vi "TC1001.vi"() -> ()   [LabVIEW 2019]
panel:
  out "ACANMsgBuffer":T1(array[cluster])
  out "初始化的数组 2":T1(array[cluster])
  out "Message&ID":string[](array[string])
  in  "发送":bool
  out "初始化的数组":string[](array[string])
  out "ALLName":string[](array[string])
  out "SignalName":string[][](array[string])
  out "Message":string[](array[string])
  in  "选项卡控件":enum32{"CANUI", "DBCUI"}(tab)
  in  "数据":T2 {"Data7" format="%x"; "Data6" format="%x"; "Data5" format="%x"; "Data4" format="%x"; "Data3" format="%x"; "Data2" format="%x"; "Data1" format="%x"; "Data0" format="%.0x"}
  in  "长度":u8
  in  "帧类型":u8(ring) items=["数据帧", "远程帧"]
  in  "帧格式":u8(ring) items=["标准帧", "扩展帧"]
  in  "ID 2":i32 format="%x"
  in  "通道选择":u8(ring) items=["CHN1", "CHN2", "CHN3", "CHN4", "CHN5", "CHN6", "CHN7", "CHN8", "CHN9", "CHN10", "CHN11", "CHN12", "CHN13", "CHN14", "CHN15", "CHN16", "CHN17", "CHN18", "CHN19", "CHN20", "CHN21", "CHN22", "CHN23", "CHN24", "CHN25", "CHN26", "CHN27", "CHN28", "CHN29", "CHN30", "CHN31", "CHN32"]
  in  "Data":i32(listbox)=-1
  in  "READ":i32(listbox)
  in  "树形控件":string(tree)
  in  "DBC路径":path
  in  "DBC加载通道":i32(ring) items=["CHN1", "CHN2", "CHN3", "CHN4", "CHN5", "CHN6", "CHN7", "CHN8", "CHN9", "CHN10", "CHN11", "CHN12", "CHN13", "CHN14", "CHN15", "CHN16", "CHN17", "CHN18", "CHN19", "CHN20", "CHN21", "CHN22", "CHN23", "CHN24", "CHN25", "CHN26", "CHN27", "CHN28", "CHN29", "CHN30", "CHN31", "CHN32"]
  in  "WRITE":string[][](table)
  out "ID":i32[](array[numeric]) format="%x"
  out "通讯":bool
  in  "波特率设置":dbl=500.0 format="%#_g k"
  in  "应用程序逻辑通道":i32(ring) items=["CHN1", "CHN2", "CHN3", "CHN4", "CHN5", "CHN6", "CHN7", "CHN8", "CHN9", "CHN10", "CHN11", "CHN12", "CHN13", "CHN14", "CHN15", "CHN16", "CHN17", "CHN18", "CHN19", "CHN20", "CHN21", "CHN22", "CHN23", "CHN24", "CHN25", "CHN26", "CHN27", "CHN28", "CHN29", "CHN30", "CHN31", "CHN32"]
  in  "物理通道":i32(ring) items=["CHN1", "CHN2", "CHN3", "CHN4", "CHN5", "CHN6", "CHN7", "CHN8", "CHN9", "CHN10", "CHN11", "CHN12", "CHN13", "CHN14", "CHN15", "CHN16", "CHN17", "CHN18", "CHN19", "CHN20", "CHN21", "CHN22", "CHN23", "CHN24", "CHN25", "CHN26", "CHN27", "CHN28", "CHN29", "CHN30", "CHN31", "CHN32"]
  in  "内置终端电阻":u16(ring)=1 items=["Disable", "Enable"]
  in  "CAN工作模式":u16(ring) items=["Normal", "ListenOnly"]
  in  "硬件型号":i32(ring)=3 items=["BUS_UNKNOWN_TYPE", "TSCANLINPro", "TSCANLINLite", "TC1001", "TL1001", "TC1011", "TM5011", "TSCAN_LITE_2", "TC1014", "TS_Reserved", "TC1026", "TC1016"]
  in  "使用通道数量":u16(ring)=1 items=["1通道"=1, "2通道"=2, "3通道"=3, "4通道"=4, "5通道"=5]
  in  "读取报文类型":u16(ring)=1 items=["只读取接收报文", "接收报文&发送报文"]
  in  "硬件启闭":bool
  in  "退出程序":bool
  # "CAN DEMO_TC1001"
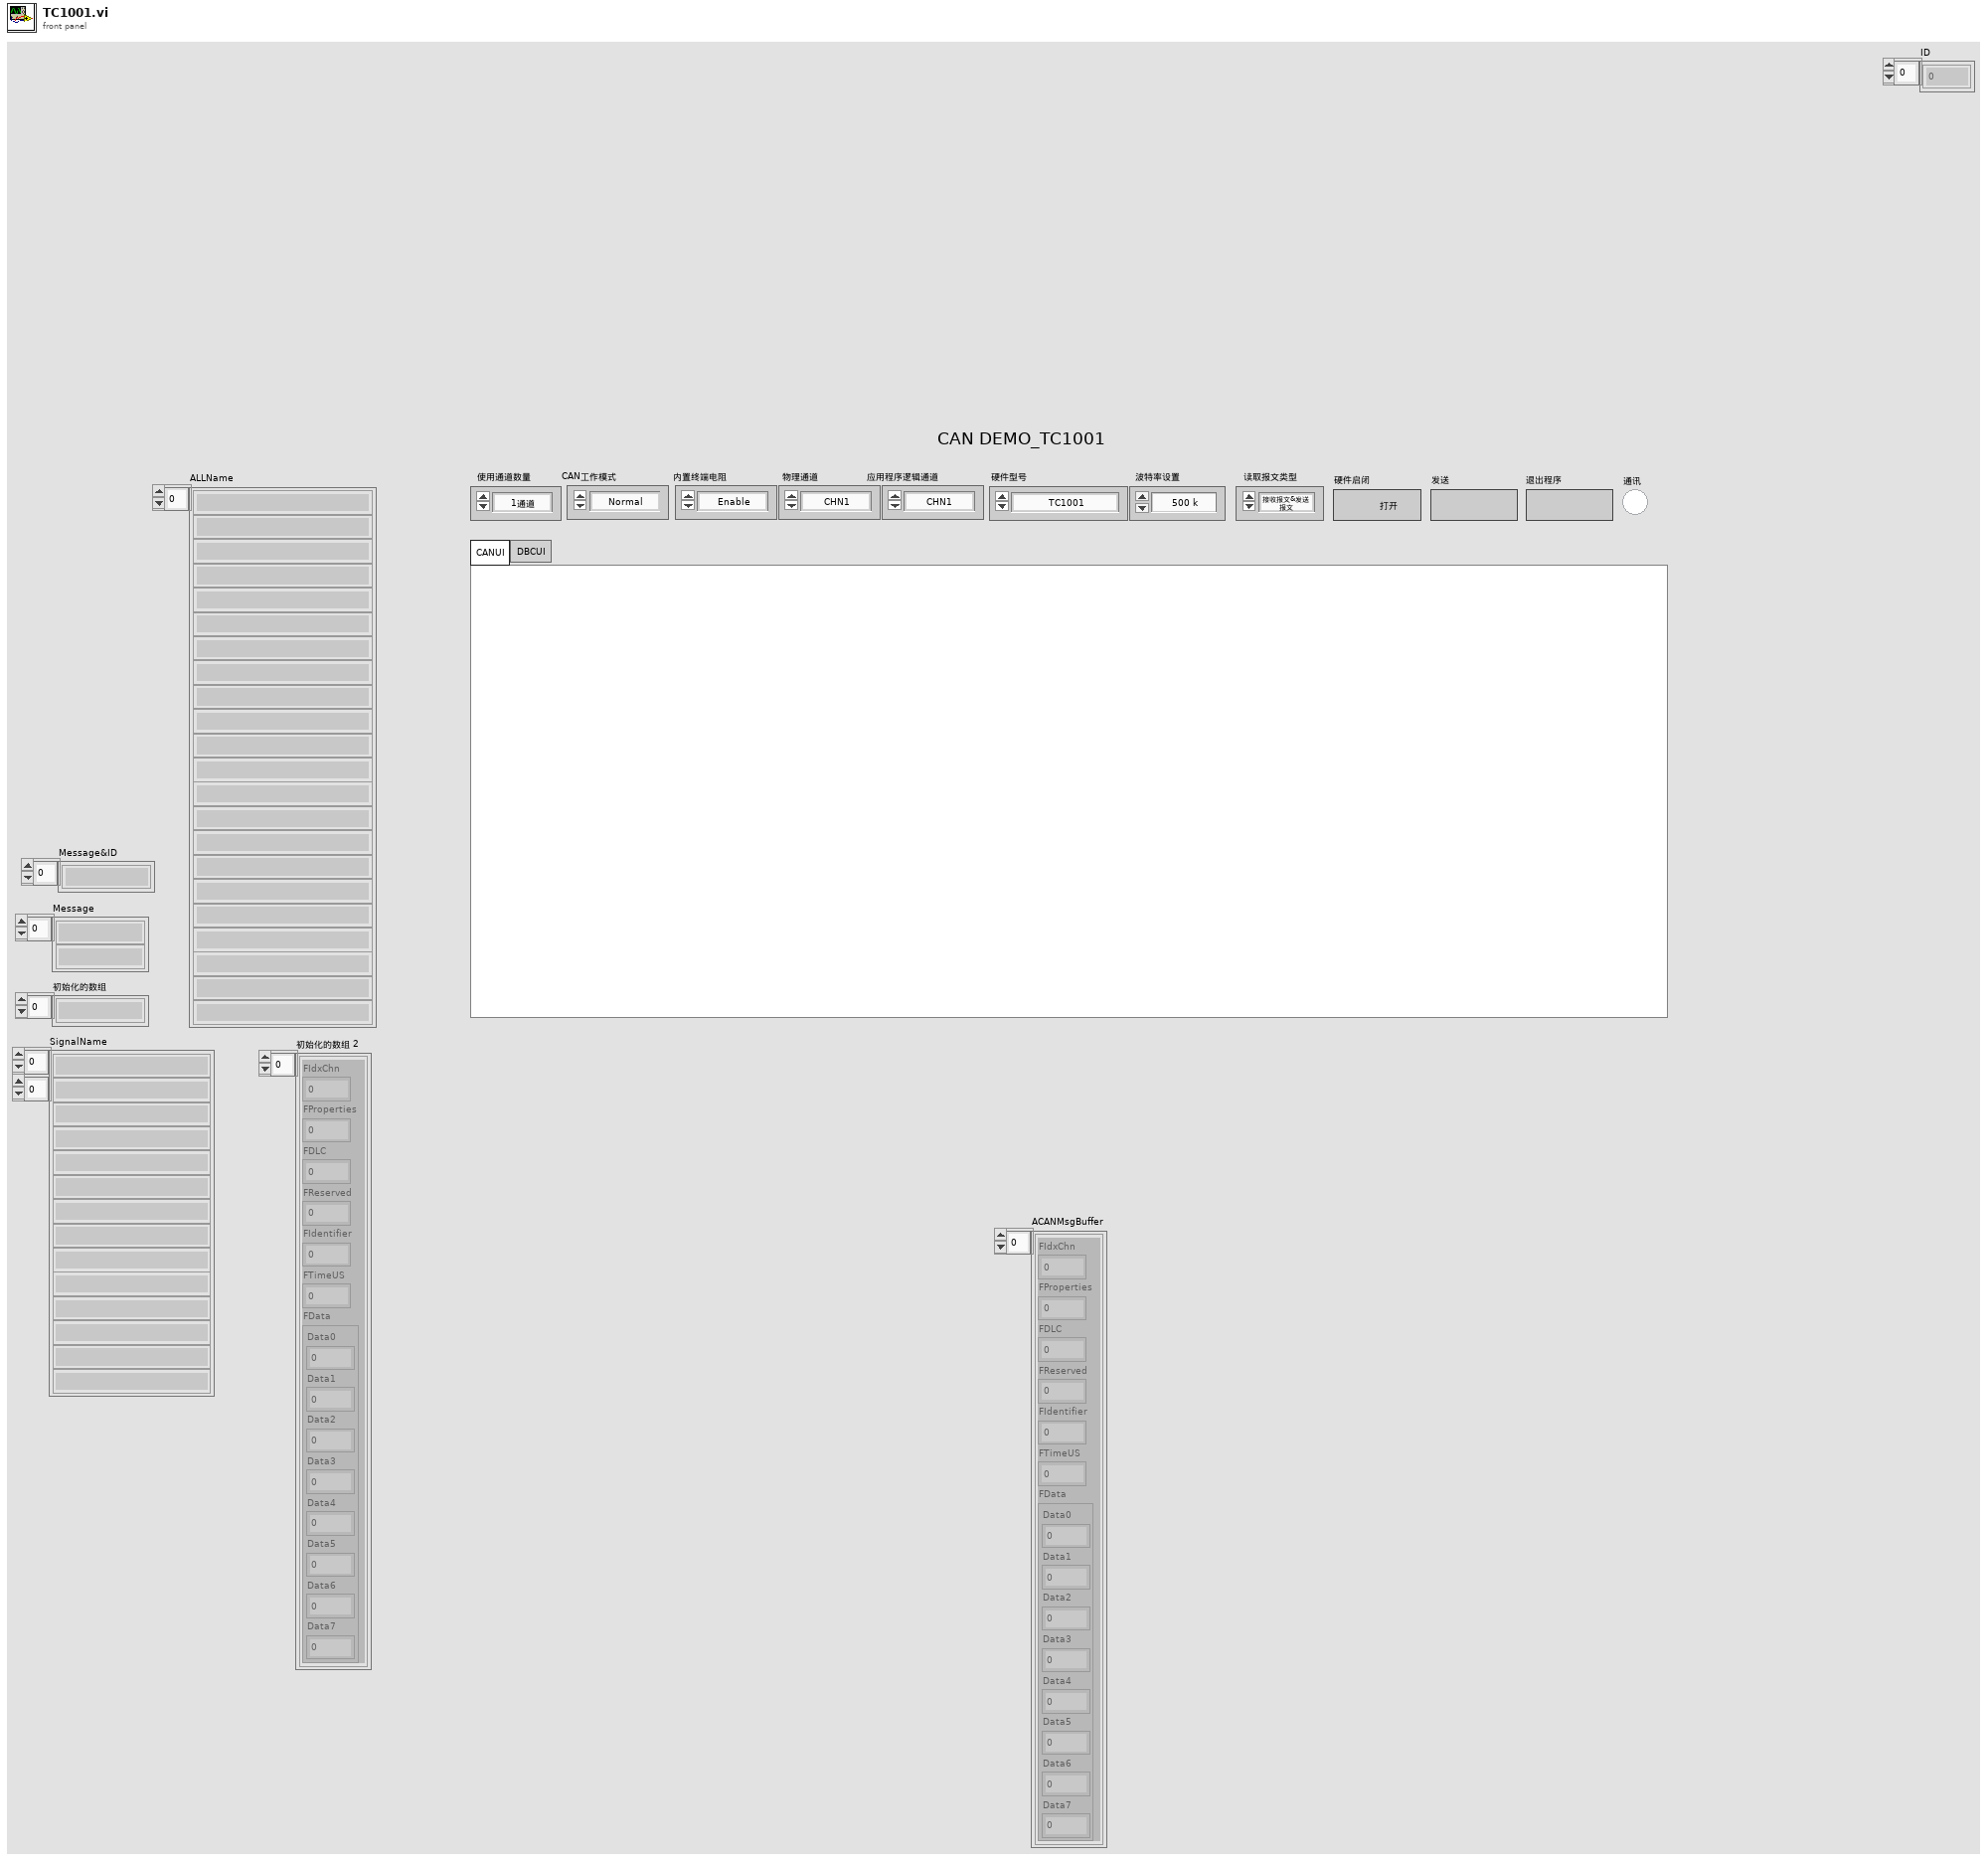
[diagram p1: front panel]
types:
  T1 = cluster{"FIdxChn":u8, "FProperties":u8, "FDLC":u8, "FReserved":u8, "FIdentifier":i32, "FTimeUS":u64, "FData":cluster{"Data0":u8, "Data1":u8, "Data2":u8, "Data3":u8, "Data4":u8, "Data5":u8, "Data6":u8, "Data7":u8}}[]
  T2 = cluster{"Data0":u8, "Data1":u8, "Data2":u8, "Data3":u8, "Data4":u8, "Data5":u8, "Data6":u8, "Data7":u8}
  T3 = cluster{"FIdxChn":u8, "FProperties":u8, "FDLC":u8, "FReserved":u8, "FIdentifier":i32, "FTimeUS":u64, "FData":cluster{"Data0":u8, "Data1":u8, "Data2":u8, "Data3":u8, "Data4":u8, "Data5":u8, "Data6":u8, "Data7":u8}}
  T4 = cluster{"硬件类型":i32, "硬件子类型":i32, "ABaudrateKbps":sgl, "AListenOnly":enum16{"Normal", "ListenOnly"}, "Int120Ohm":enum16{"Disable", "Enable"}, "EnableChannel":enum16{"Disable", "Enable"}, "AHwChannel":i32, "AAppChannel":i32}
  T5 = typedef "LVPoint32TypeDef.ctl" = cluster{"Horizontal":i32, "Vertical":i32}
  T6 = cluster{"通道选择":u8, "ID":i32, "帧格式":u8, "帧类型":u8, "长度":u8, "数据":cluster{"Data0":u8, "Data1":u8, "Data2":u8, "Data3":u8, "Data4":u8, "Data5":u8, "Data6":u8, "Data7":u8}}
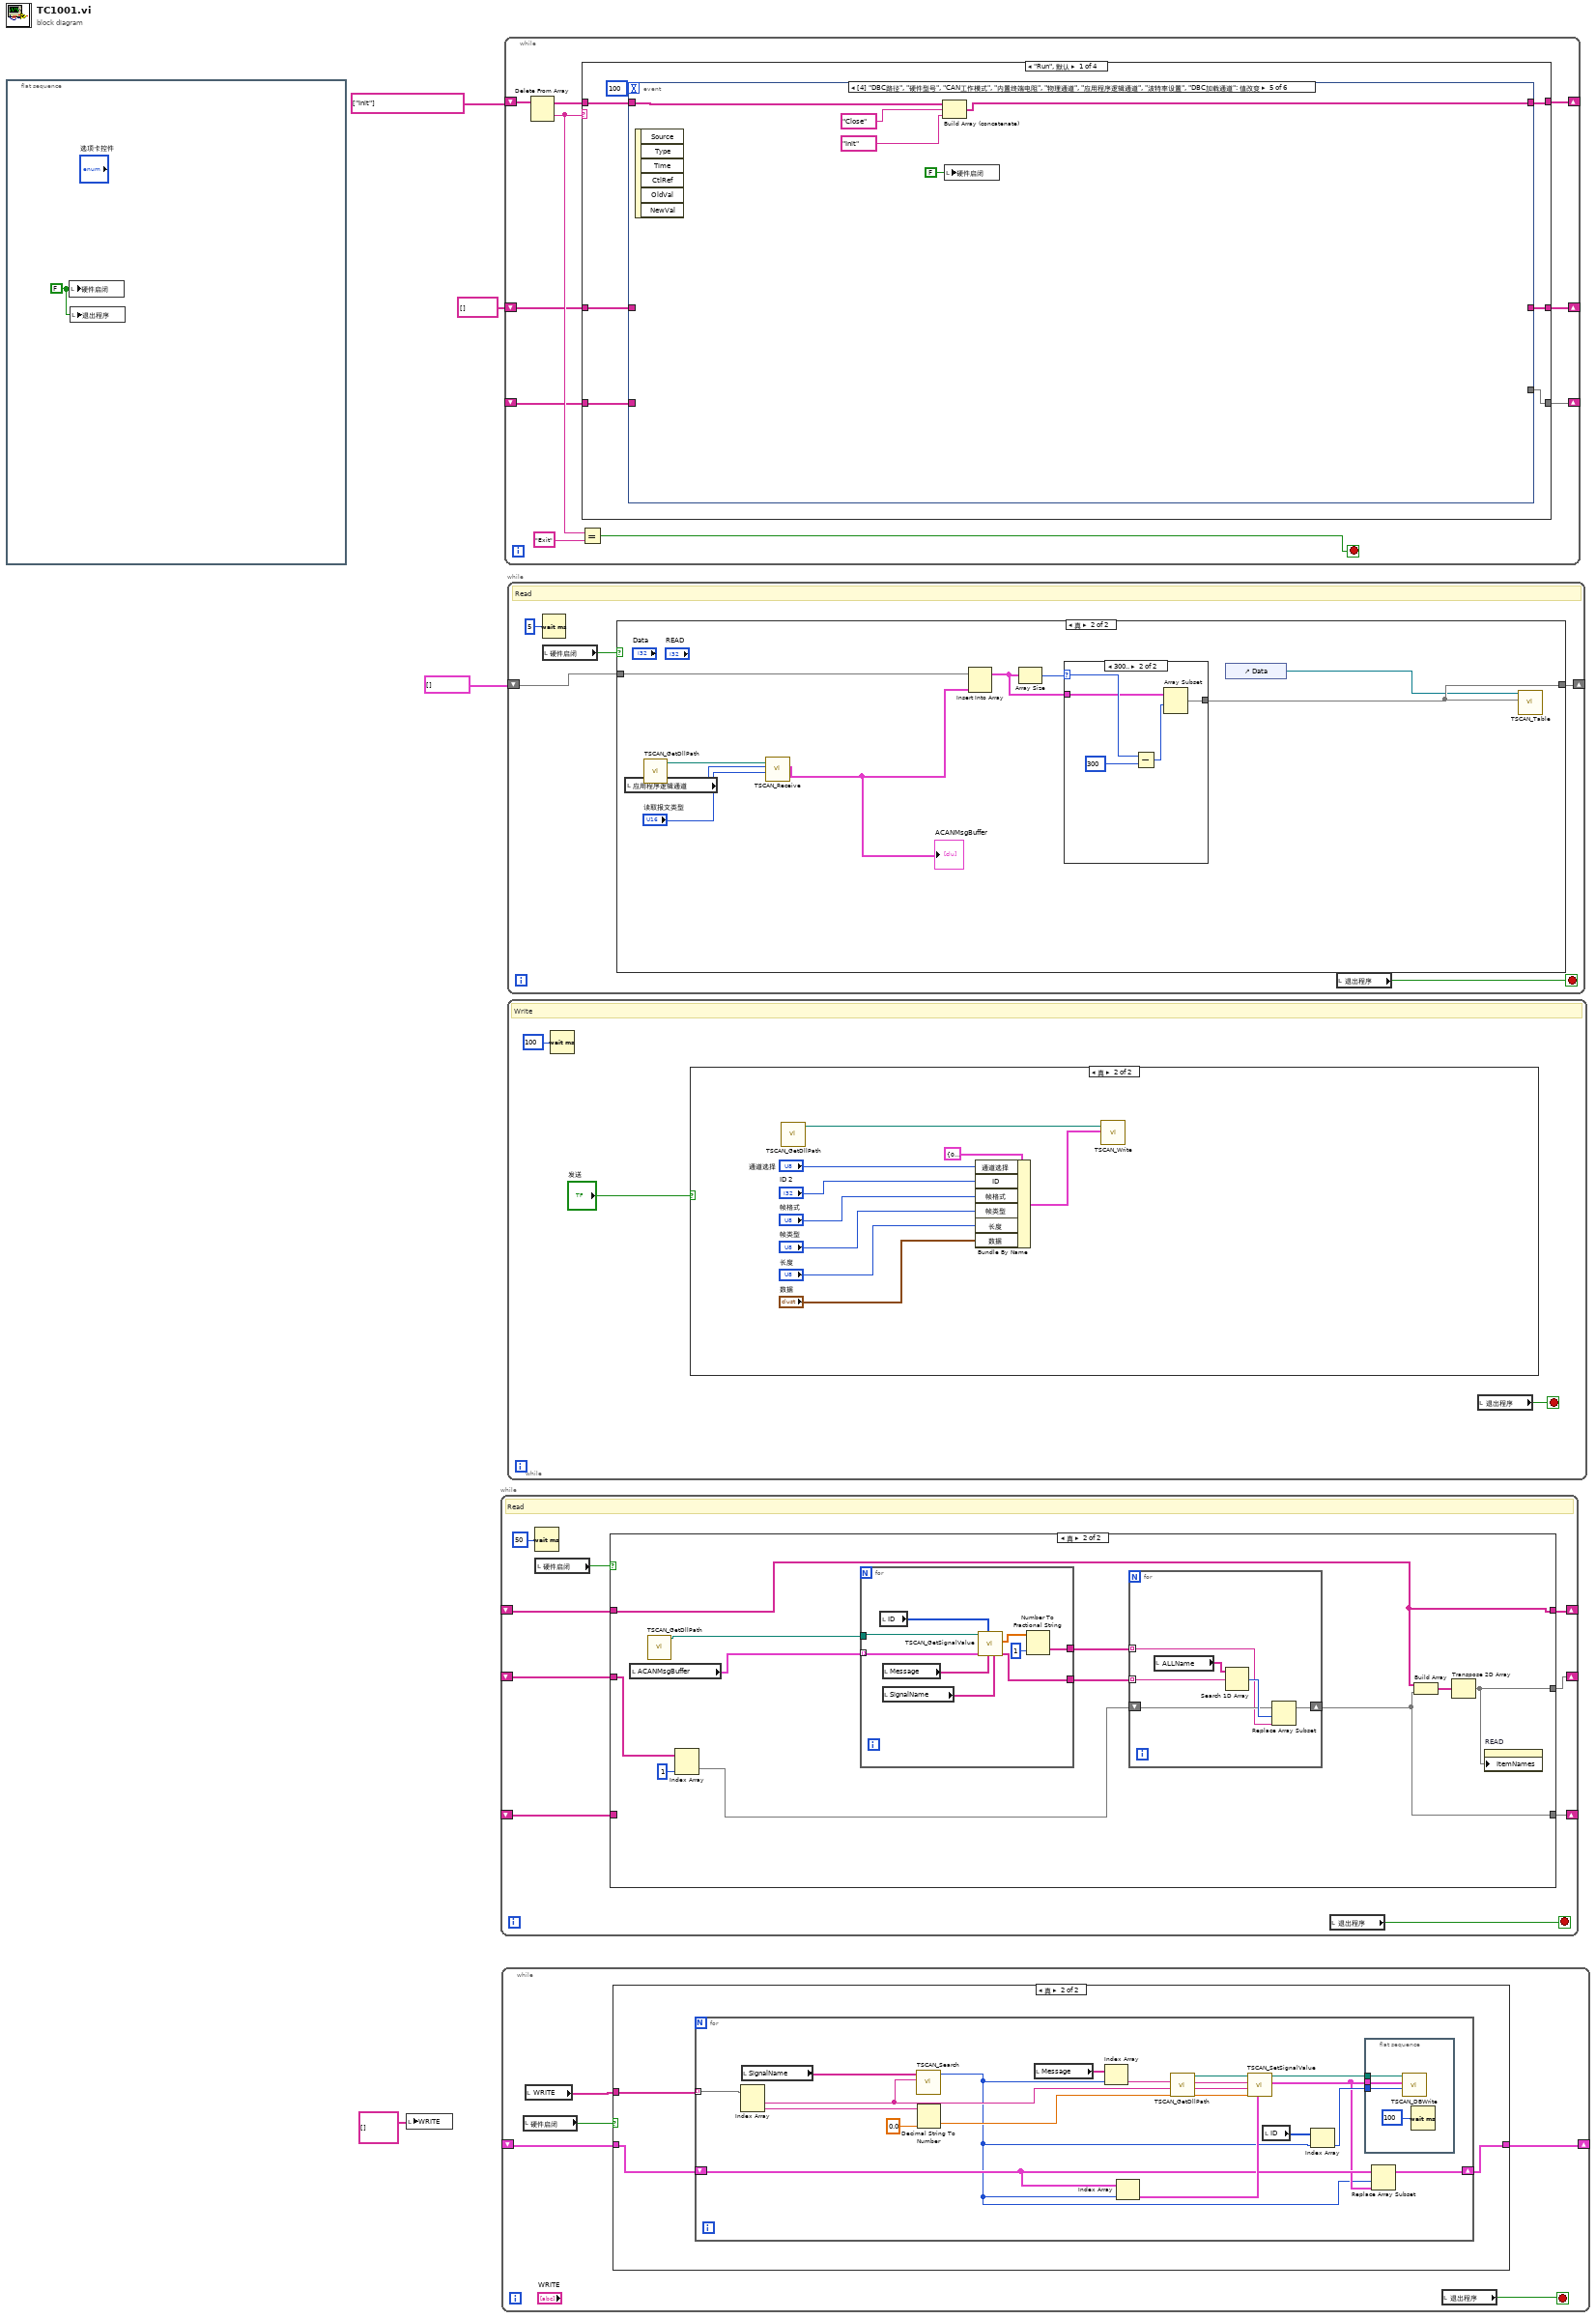
[diagram p0: block diagram]
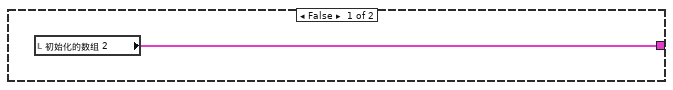
[diagram p2: hidden frame]
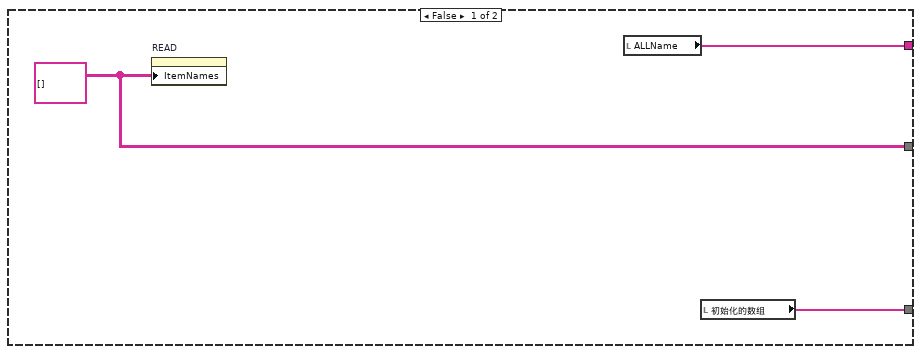
[diagram p3: hidden frame]
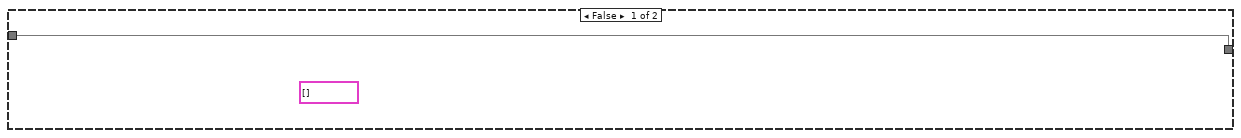
[diagram p5: hidden frame]
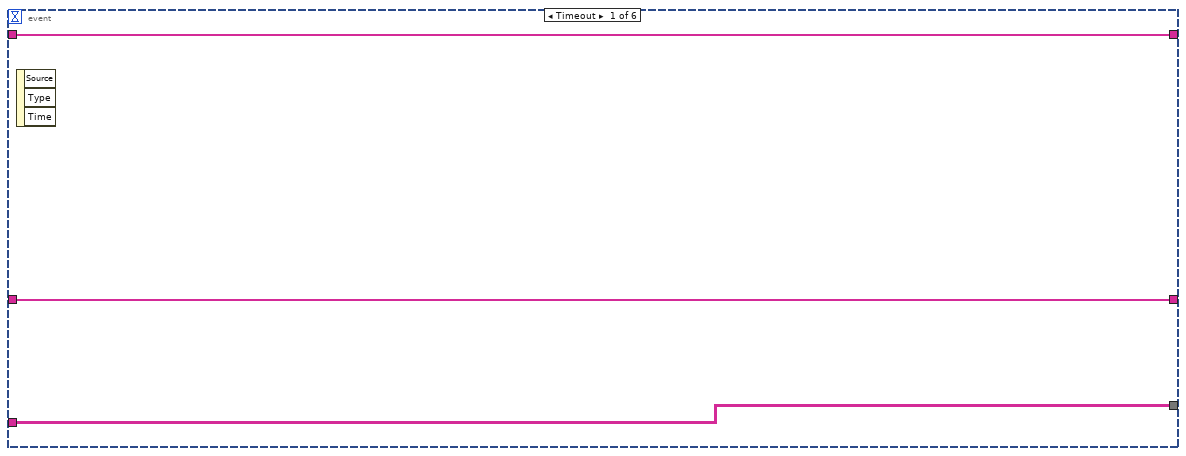
[diagram p7: hidden frame]
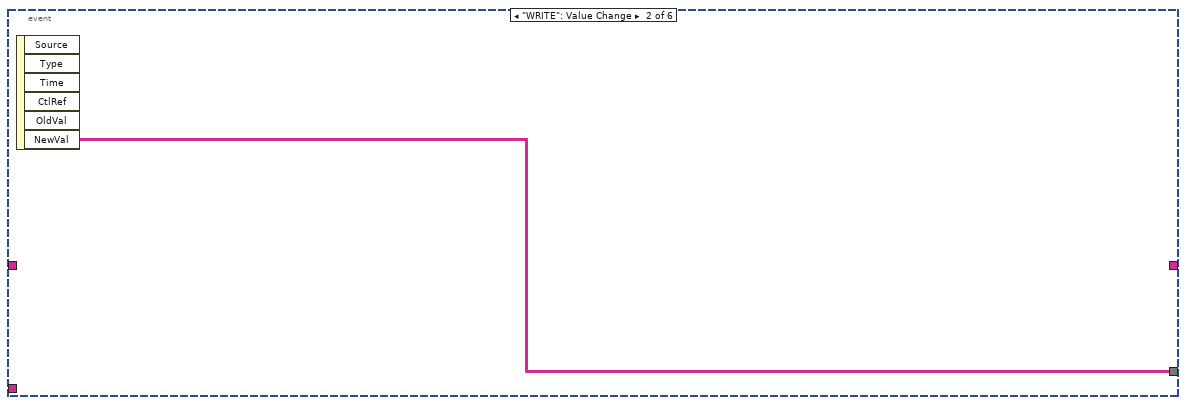
[diagram p8: hidden frame]
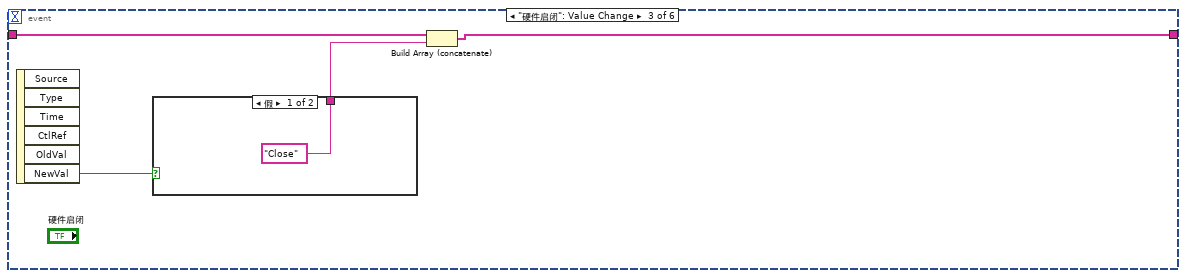
[diagram p9: hidden frame]
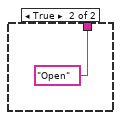
[diagram p10: hidden frame]
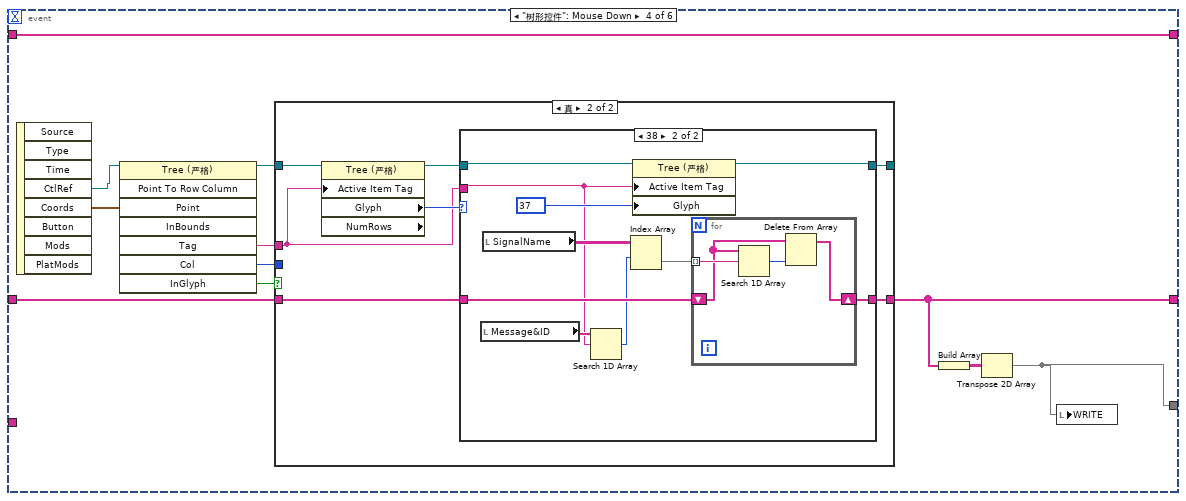
[diagram p11: hidden frame]
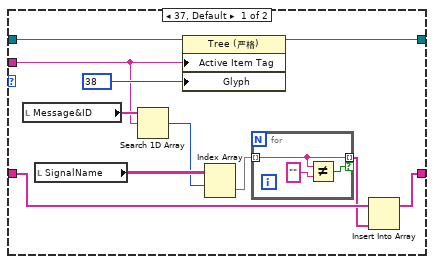
[diagram p13: hidden frame]
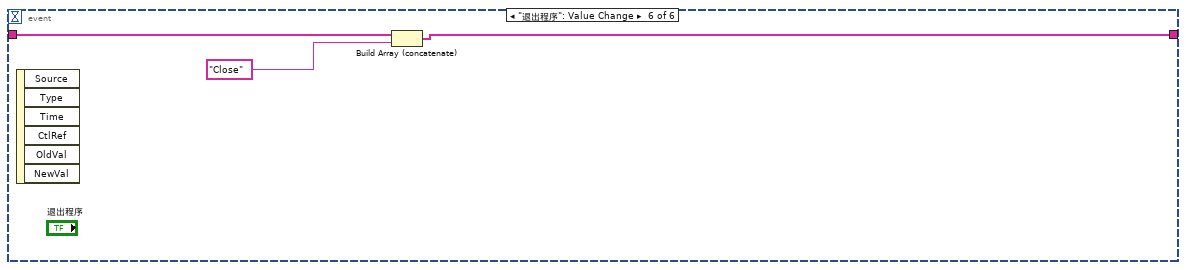
[diagram p14: hidden frame]
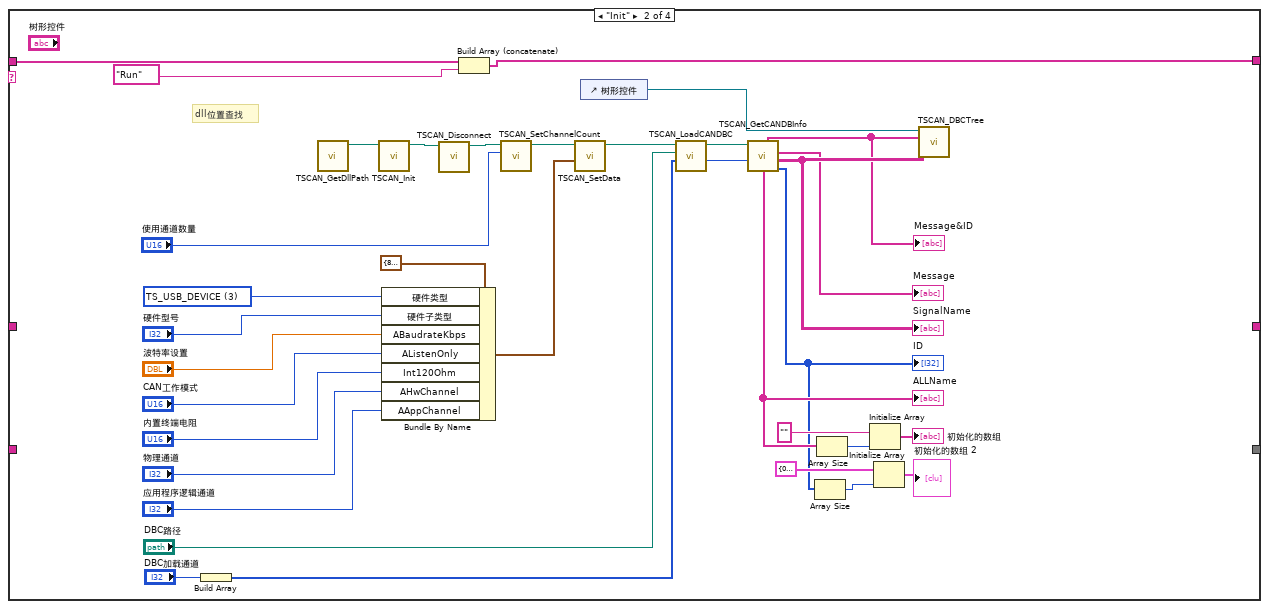
[diagram p15: hidden frame]
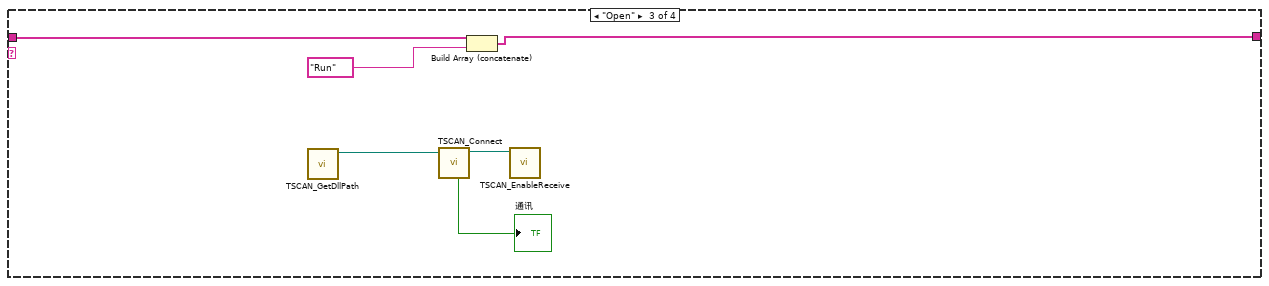
[diagram p16: hidden frame]
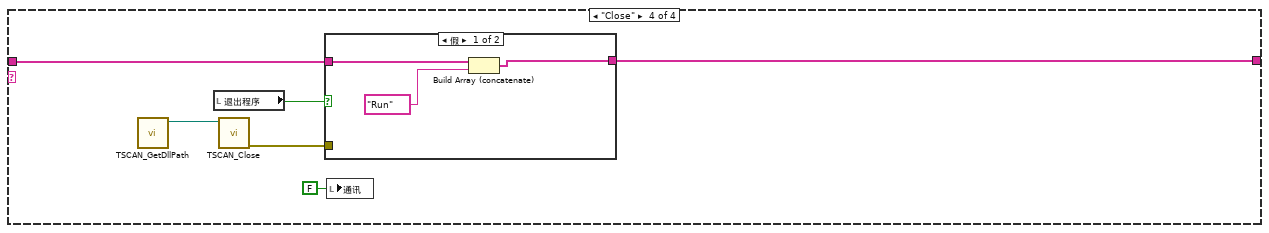
[diagram p17: hidden frame]
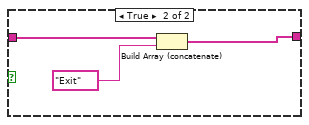
[diagram p18: hidden frame]
diagram:
  n1 = flat-sequence {
    frame #0 {
      w5 = FALSE ("硬件启闭")
      n2 = local write "硬件启闭"(w5) -> ()
      n3 = local write "退出程序"(w5) -> ()
    }
  }
  n4 = local write "WRITE"(string[][] [] ("WRITE")) -> ()
  n5 = while {
    shift-right: [w11] -> _
    shift-left: _ -> [w10]
    shift-right: [w9] -> _
    shift-left: _ -> [w8]
    shift-right: [w7] -> _
    shift-left: _ -> [w6]
    stop <- w14 stop-if-true
    # "Read"
    n6 = Wait (ms)(milliseconds to wait=u32 50 ("等待时间（毫秒）")) -> ()  [unwired: 1 out]
    n7 = local read "硬件启闭"() -> (w12:bool)
    n8 = case shown="真" w12 {
      tunnel: [w17 w24] -> w11
      tunnel: w10 -> [_ w23]
      tunnel: [w16 w25] -> w9
      tunnel: w8 -> [_ _]
      tunnel: [w15 w20] -> w7
      tunnel: w6 -> [_ w20]
      frame False {
        w17 = string[][] [] ("项名")
        n9 = property on="READ" class="MCListbox (严格)"("ItemNames"=w17) -> ()  [unwired: 2 in, 2 out]
        n10 = local read "ALLName"() -> (w15:string[])
        n11 = local read "初始化的数组"() -> (w16:string[])
      }
      frame True {
        n12 = local read "ACANMsgBuffer"() -> (w18:T1)
        n13 = call "TSCAN_GetDllPath.vi"() -> ("DllPath"=w19:path)  [unwired: 11 in]
        n14 = Index Array(array=w23, index (col)=1 ("禁用的索引 (列)")) -> (element=w21:string[])  [unwired: 1 in]
        n15 = for {
          tunnel: w19 -> [w43]
          tunnel: w18 -> [w42] mode=indexing
          tunnel: [w41] -> w27
          tunnel: [w35] -> w26
          n16 = local read "ID"() -> (w40:i32[])
          n17 = local read "Message"() -> (w39:string[])
          n18 = local read "SignalName"() -> (w38:string[][])
          n19 = call "TSCAN_GetSignalValue.vi"("ALLSignalName"=w38, "ALLMessage"=w39, "ALLID"=w40, "簇"=w42, "路径输入"=w43) -> ("数组"=w41:string[], "SigValue"=w37:dbl[])  [unwired: 3 in, 2 out]
          n20 = Number To Fractional String(number=w37, precision (6)=i16 1 ("精度(6)")) -> (F-format string=w35:string[])  [unwired: 2 in]
        }
        n21 = for {
          tunnel: w27 -> [w34] mode=indexing
          tunnel: w26 -> [w30] mode=indexing
          shift-right: [w29] -> w25
          shift-left: w21 -> [w31]
          n22 = local read "ALLName"() -> (w33:string[])
          n23 = Search 1D Array(1D array=w33, element=w34) -> (index of element=w32:i32)  [unwired: 1 in]
          n24 = Replace Array Subset(array=w31, new element=w30, index=w32) -> (w29:string[])
        }
        n25 = Build Array(w20, w25) -> (w28:string[][])
        n26 = Transpose 2D Array(2D array=w28) -> (transposed array=w24:string[][])
        n27 = property on="READ" class="MCListbox (严格)"("ItemNames"=w24) -> ()  [unwired: 2 in, 2 out]
      }
    }
    n28 = local read "退出程序"() -> (w14:bool)
  }
  n29 = while {
    shift-right: [w46] -> _
    shift-left: _ -> [w45]
    stop <- w48 stop-if-true
    n30 = local read "硬件启闭"() -> (w47:bool)
    n31 = local read "WRITE"() -> (w44:string[][])
    n32 = case shown="真" w47 {
      tunnel: [w49 w51] -> w46
      tunnel: w45 -> [_ w52]
      tunnel: w44 -> [_ w50]
      frame False {
        n33 = local read "初始化的数组 2"() -> (w49:T1)
      }
      frame True {
        n34 = for {
          tunnel: w50 -> [w68] mode=indexing
          shift-right: [w54] -> w51
          shift-left: w52 -> [w56]
          n35 = Index Array(array=w68) -> (element #1=w58:string, element #2=w65:string)  [unwired: 2 in]
          n36 = local read "SignalName"() -> (w59:string[][])
          n37 = call "TSCAN_Search.vi"("字符串"=w58, "数组"=w59) -> ("数值"=w53:i32)  [unwired: 9 in]
          n38 = Decimal String To Number(string=w65, default (0L)=0.0 ("默认(0 I32)")) -> (number=w63:dbl)  [unwired: 1 in, 1 out]
          n39 = local read "Message"() -> (w67:string[])
          n40 = Index Array(array=w67, index=w53) -> (element=w66:string)
          n41 = Index Array(array=w56, index=w53) -> (element=w57:T3)
          n42 = call "TSCAN_GetDllPath.vi"() -> ("DllPath"=w69:path)  [unwired: 11 in]
          n43 = call "TSCAN_SetSignalValue.vi"("簇"=w57, "SigValue"=w63, "Signal"=w58, "Message"=w66, "路径输入"=w69) -> ("CANObJ"=w55:T3, "路径输出"=w62:path)  [unwired: 5 in]
          n44 = local read "ID"() -> (w61:i32[])
          n45 = Index Array(array=w61, index=w53) -> (element=w60:i32)
          n46 = flat-sequence {
            tunnel: w62 -> [w73]
            tunnel: w60 -> [w72]
            tunnel: w55 -> [w71]
            frame #0 {
              n47 = call "TSCAN_DBWrite.vi"("AId"=w72, "簇"=w71, "路径输入"=w73) -> ()  [unwired: 7 in, 2 out]
              n48 = Wait (ms)(milliseconds to wait=u32 100 ("等待时间（毫秒）")) -> ()  [unwired: 1 out]
            }
          }
          n49 = Replace Array Subset(array=w56, new element=w55, index=w53) -> (w54:T1)
        }
      }
    }
    n50 = local read "退出程序"() -> (w48:bool)
  }
  n51 = while {
    shift-right: [w81] -> _
    shift-left: string[] ["Init"] -> [w83]
    shift-right: [w76] -> _
    shift-left: string[] [] -> [w77]
    shift-right: [w74] -> _
    shift-left: _ -> [w75]
    stop <- w78 stop-if-true
    n52 = Delete From Array(array=w83) -> (deleted portion=w80:string, array with subset deleted=w82:string[])  [unwired: 2 in]
    n53 = Equal?(x=w80, y="Exit") -> (x = y?=w78:bool)
    n54 = case shown="\"Run\", 默认" w80 {
      tunnel: w82 -> [w89 w190 w194 w201]
      tunnel: [w88 w189 w193 w202] -> w81
      tunnel: w77 -> [w87 _ _ _]
      tunnel: [w86 _ _ _] -> w76
      tunnel: w75 -> [w85 _ _ _]
      tunnel: [w84 _ _ _] -> w74
      frame "Run", Default {
        n55 = event shown="[4] \"DBC路径\", \"硬件型号\", \"CAN工作模式\", \"内置终端电阻\", \"物理通道\", \"应用程序逻辑通道\", \"波特率设置\", \"DBC加载通道\": 值改变" {
          selector: _ -> [_ _ _ _ _ _]
          dyn-events: _ -> [_ _ _ _ _ _]
          timeout: 100 -> [_ _ _ _ _ _]
          tunnel: w89 -> [w93 _ w98 w108 w153 w155]
          tunnel: [w93 _ w97 w108 w151 w154] -> w88
          tunnel: w87 -> [w92 _ _ w107 _ _]
          tunnel: [w92 _ _ w104 _ _] -> w86
          tunnel: w85 -> [w91 _ _ _ _ _]
          tunnel: [w91 w94 _ w101 _ _] -> w84
          event Timeout {
            n56 = event-data() -> ()  [unwired: 1 in, 3 out]
          }
          event "WRITE": Value Change {
            n57 = event-data() -> ("NewVal"=w94:string[][])  [unwired: 1 in, 5 out]
          }
          event "硬件启闭": Value Change {
            n58 = event-data() -> ("NewVal"=w96:bool)  [unwired: 1 in, 5 out]
            n59 = case shown="假" w96 {
              tunnel: ["Close" "Open"] -> w95
              frame False {
              }
              frame True {
              }
            }
            n60 = Build Array (concatenate)(w98, w95) -> (w97:string[])
          }
          event "树形控件": Mouse Down {
            n61 = event-data() -> ("CtlRef"=w102:refnum<vi>, "Coords"=w109:T5)  [unwired: 1 in, 6 out]
            n62 = invoke class="Tree (严格)" method="Point To Row Column"(reference=w102, "Point"=w109) -> (reference out=w110:refnum<vi>, "Tag"=w106:string, "Col"=w105:i32, "InGlyph"=w111:bool)  [unwired: 6 in, 4 out]
            n63 = case shown="真" w111 {
              tunnel: w106 -> [_ w117]
              tunnel: w110 -> [w113 w120]
              tunnel: [w113 w116] -> _
              tunnel: w107 -> [w112 w115]
              tunnel: [w112 w114] -> w104
              tunnel: w105 -> [_ _]
              frame False {
              }
              frame True {
                n64 = property class="Tree (严格)" props=["Active Item Tag", "Glyph", "NumRows"](reference=w120, "Active Item Tag"=w117) -> (reference out=w118:refnum<vi>, "Glyph"=w119:i32)  [unwired: 1 in, 2 out]
                n65 = case shown="38" w119 {
                  tunnel: w118 -> [w127 w143]
                  tunnel: w117 -> [w125 w136]
                  tunnel: [w131 w142] -> w116
                  tunnel: w115 -> [w123 w140]
                  tunnel: [w129 w138] -> w114
                  frame 37, Default {
                    n66 = local read "Message&ID"() -> (w126:string[])
                    n67 = local read "SignalName"() -> (w130:string[][])
                    n68 = Search 1D Array(1D array=w126, element=w125) -> (index of element=w124:i32)  [unwired: 1 in]
                    n69 = property class="Tree (严格)"(reference=w127, "Active Item Tag"=w125, "Glyph"=38) -> (reference out=w131:refnum<vi>)  [unwired: 1 in, 1 out]
                    n70 = Index Array(array=w130, index (row)=w124) -> (element=w122:string[])  [unwired: 1 in]
                    n71 = for {
                      tunnel: w122 -> [w133] mode=indexing
                      tunnel: [w133] -> w121 mode=indexing if=w134
                      n72 = Not Equal?(x=w133, y="") -> (x != y?=w134:bool)
                    }
                    n73 = Insert Into Array(array=w123, new element=w121) -> (w129:string[])  [unwired: 1 in]
                  }
                  frame 38 {
                    n74 = local read "Message&ID"() -> (w137:string[])
                    n75 = local read "SignalName"() -> (w141:string[][])
                    n76 = Search 1D Array(1D array=w137, element=w136) -> (index of element=w135:i32)  [unwired: 1 in]
                    n77 = Index Array(array=w141, index (row)=w135) -> (element=w139:string[])  [unwired: 1 in]
                    n78 = property class="Tree (严格)"(reference=w143, "Active Item Tag"=w136, "Glyph"=37) -> (reference out=w142:refnum<vi>)  [unwired: 1 in, 1 out]
                    n79 = for {
                      shift-right: [w145] -> w138
                      shift-left: w140 -> [w146]
                      tunnel: w139 -> [w148] mode=indexing
                      n80 = Search 1D Array(1D array=w146, element=w148) -> (index of element=w147:i32)  [unwired: 1 in]
                      n81 = Delete From Array(array=w146, index=w147) -> (array with subset deleted=w145:string[])  [unwired: 1 in, 1 out]
                    }
                  }
                }
              }
            }
            n82 = Build Array(w104) -> (w103:string[][])
            n83 = Transpose 2D Array(2D array=w103) -> (transposed array=w101:string[][])
            n84 = local write "WRITE"(w101) -> ()
          }
          event "DBC路径", "硬件型号", "CAN工作模式", "内置终端电阻", "物理通道", "应用程序逻辑通道", "波特率设置", "DBC加载通道": Value Change {
            n85 = event-data() -> ()  [unwired: 1 in, 6 out]
            n86 = Build Array (concatenate)(w153, "Close", "Init") -> (w151:string[])
            n87 = local write "硬件启闭"(FALSE ("硬件启闭")) -> ()
          }
          event "退出程序": Value Change {
            n88 = event-data() -> ()  [unwired: 1 in, 6 out]
            n89 = Build Array (concatenate)(w155, "Close") -> (w154:string[])
          }
        }
      }
      frame "Init" {
        w163 = 3 items=["BUS_UNKNOWN_TYPE", "TS_TCP_DEVICE", "XL_USB_DEVICE", "TS_USB_DEVICE", "PEAK_USB_DEVICE", "KVASER_USB_DEVICE", "ZLG_USB_DEVICE", "ICS_USB_DEVICE", "TS_TC1005_DEVICE"] ("硬件类型")
        # "dll位置查找"
        n90 = Build Array("DBC加载通道") -> (w185:i32[])
        n91 = call "TSCAN_GetDllPath.vi"() -> ("DllPath"=w167:path)  [unwired: 11 in]
        n92 = call "TSCAN_Init.vi"("路径输入"=w167) -> ("路径输出"=w168:path)  [unwired: 8 in, 2 out]
        n93 = Bundle By Name(cluster=T4 {"硬件类型"=8, "硬件子类型"=0, "ABaudrateKbps"=250.0, "AListenOnly"=enum."Normal", "Int120Ohm"=enum."Enable", "EnableChannel"=enum."Enable", "AHwChannel"=0, "AAppChannel"=0} ("CAN配置"), "硬件类型"=w163, "硬件子类型"="硬件型号", "ABaudrateKbps"="波特率设置", "AListenOnly"="CAN工作模式", "Int120Ohm"="内置终端电阻", "AHwChannel"="物理通道", "AAppChannel"="应用程序逻辑通道") -> (w164:T4)
        n94 = call "TSCAN_Disconnect.vi"("路径输入"=w168) -> ("路径输出"=w169:path)  [unwired: 9 in, 1 out]
        n95 = Build Array (concatenate)(w190, "Run") -> (w189:string[])
        n96 = call "TSCAN_SetChannelCount.vi"("Aount"="使用通道数量", "路径输入"=w169) -> ("路径输出"=w170:path)  [unwired: 7 in, 2 out]
        n97 = call "TSCAN_SetData.vi"("CAN配置"=w164, "路径输入"=w170) -> ("路径输出"=w188:path)  [unwired: 5 in, 4 out]
        n98 = control-ref of="树形控件"() -> (w182:refnum<vi>)
        n99 = call "TSCAN_LoadCANDBC.vi"("ABindChannels"=w185, "ADBCAbsolutePath"="DBC路径", "路径输入"=w188) -> ("AIdOut"=w183:u32, "路径输出"=w184:path)  [unwired: 5 in, 2 out]
        n100 = call "TSCAN_GetCANDBInfo.vi"("ADatabaseld"=w183, "路径输入"=w184) -> ("ID"=w172:i32[], "SignalName"=w181:string[][], "Message"=→"Message":string[], "Message&ID"=w180:string[], "ALLName"=w177:string[])  [unwired: 3 in, 1 out]
        "ID" <- w172
        "SignalName" <- w181
        "ALLName" <- w177
        "Message&ID" <- w180
        n101 = Array Size(array=w172) -> (size(s)=w173:i32)
        n102 = Array Size(array=w177) -> (size(s)=w178:i32)
        n103 = Initialize Array("", w178) -> (→"初始化的数组":string[])
        n104 = Initialize Array(T3 {"FIdxChn"=0, "FProperties"=0, "FDLC"=0, "FReserved"=0, "FIdentifier"=0, "FTimeUS"=0, "FData"={"Data0"=0, "Data1"=0, "Data2"=0, "Data3"=0, "Data4"=0, "Data5"=0, "Data6"=0, "Data7"=0}} ("CANObJ"), w173) -> (→"初始化的数组 2":T1)
        n105 = call "TSCAN_DBCTree.vi"("子节点"=w181, "父节点"=w180, "控件"=w182) -> ()  [unwired: 9 in]
      }
      frame "Open" {
        n106 = call "TSCAN_GetDllPath.vi"() -> ("DllPath"=w196:path)  [unwired: 11 in]
        n107 = call "TSCAN_Connect.vi"("路径输入"=w196) -> ("路径输出"=w197:path, "Connect_TSCAN_Successfully"=→"通讯":bool)  [unwired: 8 in, 1 out]
        n108 = Build Array (concatenate)(w194, "Run") -> (w193:string[])
        n109 = call "TSCAN_EnableReceive.vi"("路径输入"=w197) -> ()  [unwired: 9 in, 2 out]
      }
      frame "Close" {
        n110 = call "TSCAN_GetDllPath.vi"() -> ("DllPath"=w200:path)  [unwired: 11 in]
        n111 = local read "退出程序"() -> (w203:bool)
        n112 = call "TSCAN_Close.vi"("路径输入"=w200) -> ("错误输出"=w199:errorcluster)  [unwired: 9 in, 1 out]
        n113 = case shown="假" w203 {
          tunnel: [w204 w208] -> w202
          tunnel: w201 -> [w205 w207]
          tunnel: w199 -> [_ _]
          frame False {
            n114 = Build Array (concatenate)(w205, "Run") -> (w204:string[])
          }
          frame True {
            n115 = Build Array (concatenate)(w207, "Exit") -> (w208:string[])
          }
        }
        n116 = local write "通讯"(FALSE ("通讯")) -> ()
      }
    }
  }
  n117 = while {
    stop <- w212 stop-if-true
    # "Write"
    n118 = Wait (ms)(milliseconds to wait=u32 100 ("等待时间（毫秒）")) -> ()  [unwired: 1 out]
    n119 = case shown="真" "发送" {
      frame False {
      }
      frame True {
        n120 = call "TSCAN_GetDllPath.vi"() -> ("DllPath"=w221:path)  [unwired: 11 in]
        n121 = Bundle By Name(cluster=T6 {"通道选择"=0, "ID"=274, "帧格式"=0, "帧类型"=0, "长度"=3, "数据"={"Data0"=11, "Data1"=0, "Data2"=0, "Data3"=0, "Data4"=0, "Data5"=0, "Data6"=0, "Data7"=0}} ("TCAN"), "通道选择"="通道选择", "ID"="ID 2", "帧格式"="帧格式", "帧类型"="帧类型", "长度"="长度", "数据"="数据") -> (w213:T6)
        n122 = call "TSCAN_Write.vi"("TCAN"=w213, "路径输入"=w221) -> ()  [unwired: 8 in, 2 out]
      }
    }
    n123 = local read "退出程序"() -> (w212:bool)
  }
  n124 = while {
    shift-right: [w222] -> _
    shift-left: T1 [] ("数组") -> [w223]
    stop <- w226 stop-if-true
    # "Read"
    n125 = Wait (ms)(milliseconds to wait=u32 5 ("等待时间（毫秒）")) -> ()  [unwired: 1 out]
    n126 = local read "硬件启闭"() -> (w224:bool)
    n127 = case shown="真" w224 {
      tunnel: [w227 w231] -> w222
      tunnel: w223 -> [w227 w234]
      frame False {
        (unwired) T1 [] ("数组")
      }
      frame True {
        n128 = local read "应用程序逻辑通道"() -> (w235:i32)
        n129 = call "TSCAN_GetDllPath.vi"() -> ("DllPath"=w236:path)  [unwired: 11 in]
        n130 = call "TSCAN_Receive.vi"("读取报文类型"="读取报文类型", "AAPPChannel"=w235, "路径输入"=w236) -> ("ACANMsgBuffer"=w228:T1)  [unwired: 5 in, 2 out]
        "ACANMsgBuffer" <- w228
        n131 = Insert Into Array(array=w234, new element=w228) -> (w232:T1)  [unwired: 1 in]
        n132 = Array Size(array=w232) -> (size(s)=w233:i32)
        n133 = case shown="300.." w233 {
          selector: w233 -> [_ w242]
          tunnel: [w237 w240] -> w231
          tunnel: w232 -> [w237 w238]
          frame 0, Default {
          }
          frame 300.. {
            n134 = Subtract(x=w242, y=300) -> (x-y=w239:i32)
            n135 = Array Subset(array=w238, index=w239) -> (w240:T1)  [unwired: 1 in]
          }
        }
        n136 = control-ref of="Data"() -> (w229:refnum<vi>)
        n137 = call "TSCAN_Table.vi"("Buffer"=w231, "MCListbox引用句柄"=w229) -> ()  [unwired: 10 in]
      }
    }
    n138 = local read "退出程序"() -> (w226:bool)
  }
